vi "Global-Var-Simulator.vi"() -> ()   [LabVIEW 2021]
panel:
  out "simulator_on":bool
  out "shiner_low_level_G":bool
  out "soap_low_level_G":bool
  out "water_low_level_G":bool
  out "stop_simulator":bool
  out "is_alarm_state_Wash1_G":bool
  in  "wash_mode_G":string
  out "seconds_G":dbl
  out "minutes_G":dbl
  out "shiner_level_G":dbl
  out "soap_level_G":dbl
  out "water_level_G":dbl
  out "is_running_G":bool
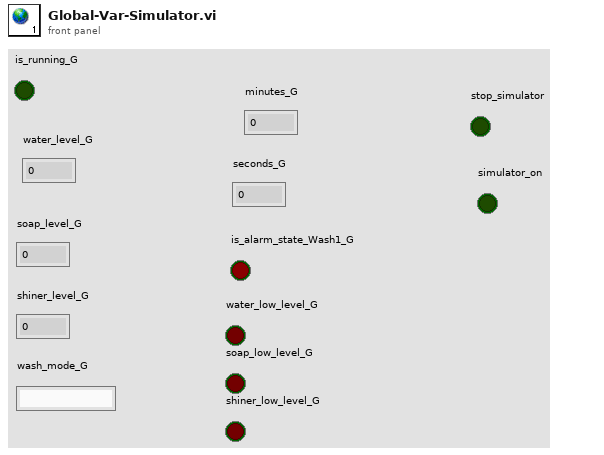
[diagram p1: front panel]
diagram:
